vi "configureStream.vi"(8 "error in (no error)":errorcluster, 11 "SoundAO in":refnum<class "SoundAO.lvclass">) -> (0 "error out":errorcluster, 3 "SoundAO out":refnum<class "SoundAO.lvclass">)   [LabVIEW 2011, in "Hardware.lvlib" / "Channels.lvlib" / "SoundAO.lvclass"]
uses:
  SoundAO.lvclass
  SoundAO.lvclass/SoundAO.ctl
  AnalogOutput.lvclass
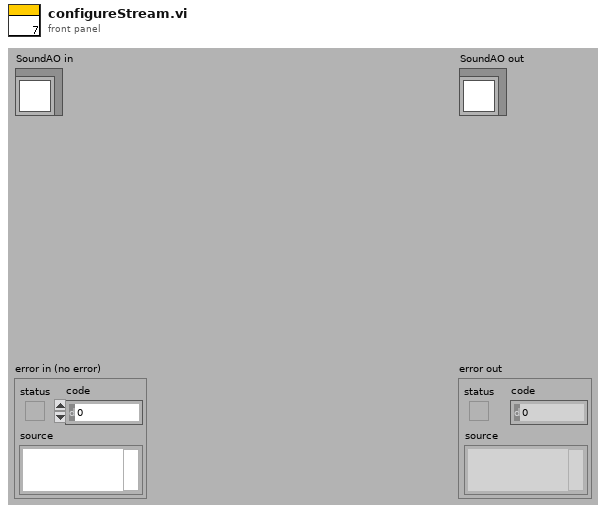
[diagram p1: front panel]
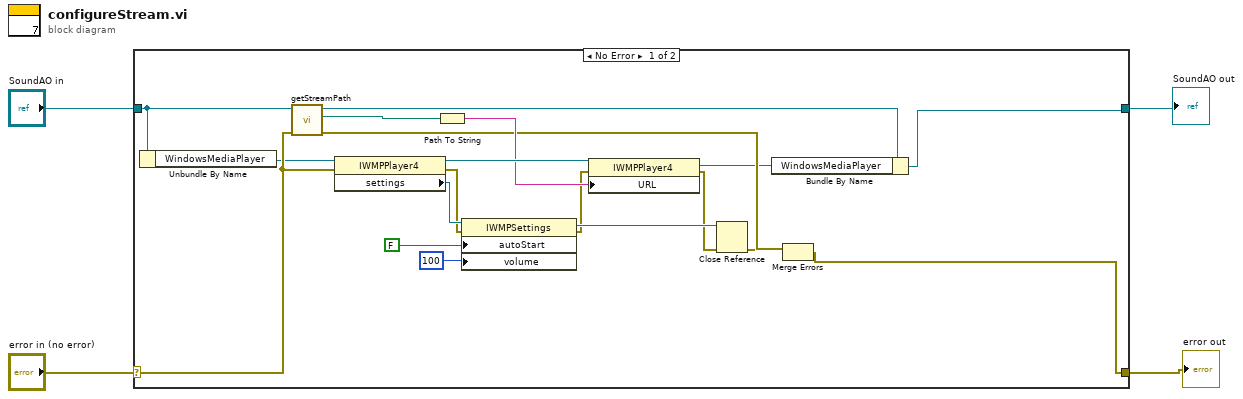
[diagram p0: block diagram]
diagram:
  n1 = case shown="No Error" "error in (no error)" {
    selector: "error in (no error)" -> [w7 w25]
    tunnel: [w5 w25] -> w3
    tunnel: [w9 w24] -> w1
    tunnel: "SoundAO in" -> [w18 w24]
    frame No Error {
      n2 = Unbundle By Name(w18) -> ("WindowsMediaPlayer"=w6:refnum<k7>)
      n3 = call "getStreamPath.vi"("error in (no error)"=w7, "AnalogOutput.lvclass in"=w18) -> ("error out"=w13:errorcluster, "streamPath"=w17:path, "AnalogOutput.lvclass out"=w10:refnum<class "SoundAO.lvclass">)  [unwired: 7 in]
      n4 = property class="IWMPPlayer4"(reference=w6, error in=w7) -> (reference out=w20:refnum<k7>, error out=w19:errorcluster, "settings"=w21:refnum<k7>)
      n5 = Path To String(path=w17) -> (string=w16:string)
      n6 = property class="IWMPSettings"(reference=w21, error in=w19, "autoStart"=FALSE, "volume"=100 ("balance")) -> (reference out=w22:refnum<k7>, error out=w15:errorcluster)
      n7 = property class="IWMPPlayer4"(reference=w20, error in=w15, "URL"=w16) -> (reference out=w11:refnum<k7>, error out=w14:errorcluster)
      n8 = Close Reference(reference=w22, error in (no error)=w14) -> (error out=w12:errorcluster)
      n9 = Bundle By Name(cluster=w10, "WindowsMediaPlayer"=w11) -> (w9:refnum<class "SoundAO.lvclass">)
      n10 = Merge Errors(w13, w12) -> (w5:errorcluster)
    }
    frame Error {
    }
  }
  "error out" <- w3
  "SoundAO out" <- w1
